vi "Construct_String.vi"(11 "Tx Data":T1) -> (3 "String":string)   [LabVIEW 2020]
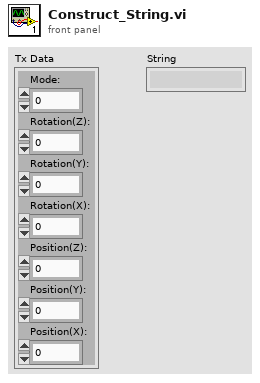
[diagram p1: front panel]
types:
  T1 = cluster{"Mode:":i32, "Rotation(Z):":dbl, "Rotation(Y):":dbl, "Rotation(X):":dbl, "Position(Z):":dbl, "Position(Y):":dbl, "Position(X):":dbl}
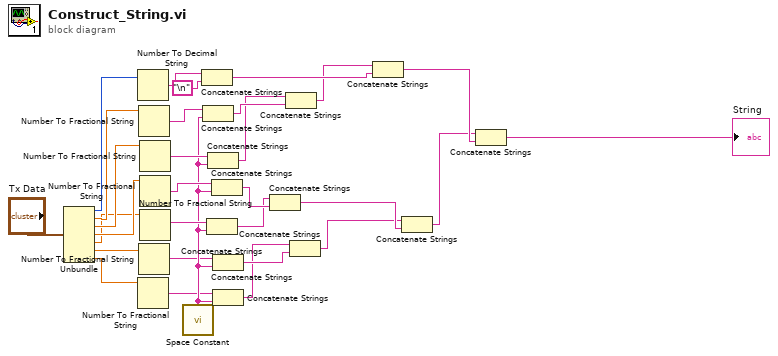
[diagram p0: block diagram]
diagram:
  n1 = Unbundle("Tx Data") -> ("Mode:"=w8:i32, "Rotation(Z):"=w7:dbl, "Rotation(Y):"=w6:dbl, "Rotation(X):"=w5:dbl, "Position(Z):"=w4:dbl, "Position(Y):"=w3:dbl, "Position(X):"=w2:dbl)
  n2 = Number To Decimal String(number=w8) -> (decimal integer string=w16:string)  [unwired: 1 in]
  n3 = Number To Fractional String(number=w2) -> (F-format string=w9:string)  [unwired: 3 in]
  n4 = Number To Fractional String(number=w7) -> (F-format string=w15:string)  [unwired: 3 in]
  n5 = Number To Fractional String(number=w3) -> (F-format string=w10:string)  [unwired: 3 in]
  n6 = Number To Fractional String(number=w6) -> (F-format string=w14:string)  [unwired: 3 in]
  n7 = Number To Fractional String(number=w5) -> (F-format string=w13:string)  [unwired: 3 in]
  n8 = Number To Fractional String(number=w4) -> (F-format string=w12:string)  [unwired: 3 in]
  n9 = call <vilib>:"Space Constant.vi"() -> ("String"=w11:string)
  n10 = Concatenate Strings(w16, "\n") -> (w24:string)
  n11 = Concatenate Strings(w15, w11) -> (w22:string)
  n12 = Concatenate Strings(w12, w11) -> (w19:string)
  n13 = Concatenate Strings(w14, w11) -> (w21:string)
  n14 = Concatenate Strings(w13, w11) -> (w20:string)
  n15 = Concatenate Strings(w10, w11) -> (w18:string)
  n16 = Concatenate Strings(w9, w11) -> (w17:string)
  n17 = Concatenate Strings(w19, w20) -> (w26:string)
  n18 = Concatenate Strings(w21, w22) -> (w23:string)
  n19 = Concatenate Strings(w17, w18) -> (w25:string)
  n20 = Concatenate Strings(w23, w24) -> (w28:string)
  n21 = Concatenate Strings(w25, w26) -> (w27:string)
  n22 = Concatenate Strings(w27, w28) -> (→"String":string)
